vi "Get Date and Time (sec).vi"(2 "error in":errorcluster) -> (0 "error out":errorcluster, 1 "seconds since 1Jan1904":timestamp)   [LabVIEW 2018]
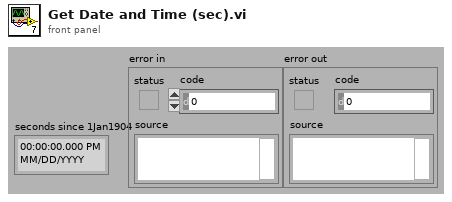
[diagram p1: front panel]
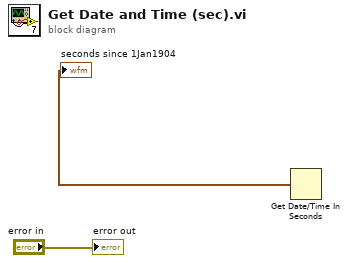
[diagram p0: block diagram]
diagram:
  n1 = Get Date/Time In Seconds() -> (seconds since 1Jan1904=→"seconds since 1Jan1904":timestamp)
  "error out" <- "error in"
